vi "oa_Create Indice Lock Finish.vi"(2 "finish?":bool, 3 "reset?(F)":bool) -> (0 "locked finish":bool)   [LabVIEW 2017, in "SoundVib_OAUtility.lvlib"]
uses:
  <vilib>/addons/Sound and Vibration/Order Analysis/Utility/SoundVib_OAUtility.lvlib
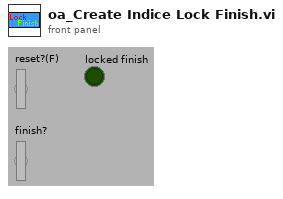
[diagram p1: front panel]
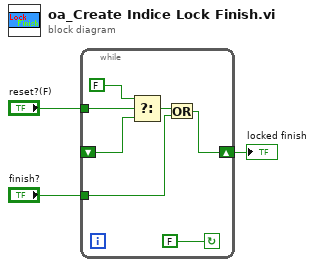
[diagram p0: block diagram]
diagram:
  n1 = while {
    tunnel: "reset?(F)" -> [w9]
    tunnel: "finish?" -> [w5]
    shift-right: [w4] -> w1
    shift-left: _ -> [w7]
    stop <- FALSE continue-if-true
    n2 = Select(t=FALSE, s=w9, f=w7) -> (s? t:f=w6:bool)
    n3 = Or(x=w6, y=w5) -> (x .or. y?=w4:bool)
  }
  "locked finish" <- w1
